vi "按日期创建文件夹按时间写入TXT.vi"() -> ()   [LabVIEW 2014]
panel:
  in  "停止":bool
  out "created path":path
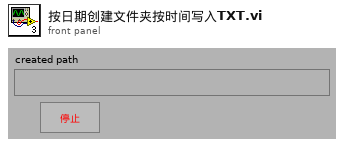
[diagram p1: front panel]
types:
  T1 = enum16{"open", "replace", "create", "open or create", "replace or create", "replace or create with confirmation"}
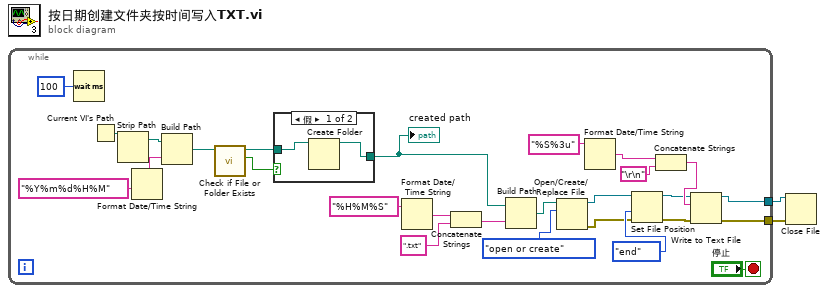
[diagram p0: block diagram]
diagram:
  n1 = while {
    tunnel: [w8] -> w2
    tunnel: [w7] -> w1
    stop <- "停止" stop-if-true
    n2 = Wait (ms)(milliseconds to wait=u32 100 ("等待时间（毫秒）")) -> ()  [unwired: 1 out]
    n3 = Current VI's Path() -> (path=w29:path)
    n4 = Strip Path(path=w29) -> (stripped path=w28:path)  [unwired: 1 out]
    n5 = Format Date/Time String(time format string (%c)="%Y%m%d%H%M" ("时间格式字符串(%c)")) -> (date/time string=w5:string)  [unwired: 2 in]
    n6 = Build Path(base path=w28, name or relative path=w5) -> (appended path=w27:path)
    n7 = call <vilib>:"Check if File or Folder Exists.vi"("path"=w27) -> ("file or folder exists?"=w25:bool, "dup path"=w26:path)  [unwired: 8 in, 1 out]
    n8 = case shown="假" w25 {
      tunnel: w26 -> [w31 w32]
      tunnel: [w30 w32] -> w3
      frame False {
        n9 = Create Folder(path (use dialog)=w31) -> (created path=w30:path)  [unwired: 2 in, 2 out]
      }
      frame True {
      }
    }
    "created path" <- w3
    n10 = Format Date/Time String(time format string (%c)="%H%M%S" ("时间格式字符串(%c)")) -> (date/time string=w16:string)  [unwired: 2 in]
    n11 = Concatenate Strings(w16, ".txt" ("字符串")) -> (w17:string)
    n12 = Build Path(base path=w3, name or relative path=w17) -> (appended path=w20:path)
    n13 = Open/Create/Replace File(file path (use dialog)=w20, operation (0:open)=T1."open or create" ("操作(0:open)")) -> (refnum out=w21:refnum<file>, error out=w22:errorcluster)  [unwired: 4 in, 1 out]
    n14 = Format Date/Time String(time format string (%c)="%S%3u" ("时间格式字符串(%c)")) -> (date/time string=w12:string)  [unwired: 2 in]
    n15 = Set File Position(refnum=w21, from (0:start)=enum16{"start", "end", "current"}."end" ("自（0:起始）"), error in=w22) -> (refnum out=w10:refnum<file>, error out=w9:errorcluster)  [unwired: 1 in]
    n16 = Concatenate Strings(w12, "\r\n") -> (w11:string)
    n17 = Write to Text File(file (use dialog)=w10, text=w11, error in=w9) -> (refnum out=w8:refnum<file>, error out=w7:errorcluster)  [unwired: 1 in, 1 out]
  }
  n18 = Close File(refnum=w2, error in=w1) -> ()  [unwired: 2 out]
